vi "1_FindWorkingZDistancewPlaceholder.vi"(6 "Axis Speeds":T2, 7 "Focusing test interval [mm]":dbl, 8 "error in (no error)":errorcluster, 9 "Stepsize [mm]":dbl, 10 "Autofocus Coordinates":T3, 11 "Session in":T1) -> (0 "error out":errorcluster, 1 "Optimized working distance":dbl, 2 "XYZ Stage Current Position":T4, 3 "Session out":T1, 5 "Finished!":bool)   [LabVIEW 2016]
uses:
  <vilib>/userdefined/High Color/IMAQdx.ctl
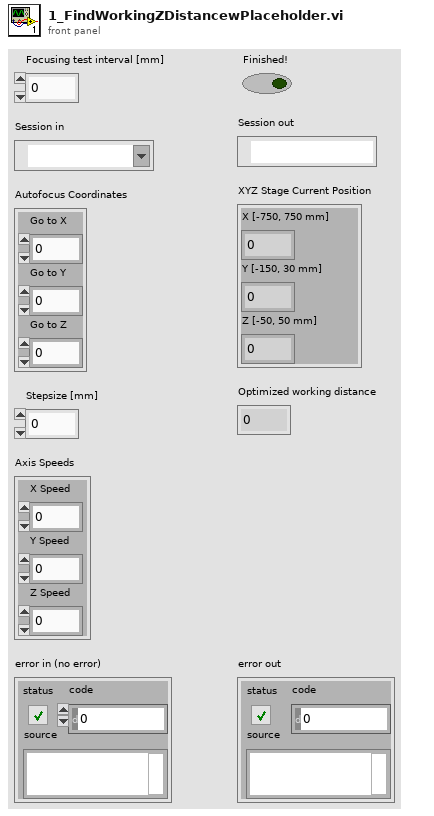
[diagram p1: front panel]
types:
  T1 = typedef "IMAQdx.ctl" = refnum<k21>
  T2 = cluster{"X Speed":dbl, "Y Speed":dbl, "Z Speed":dbl}
  T3 = cluster{"Go to X":dbl, "Go to Y":dbl, "Go to Z":dbl}
  T4 = cluster{"X [-750, 750 mm]":dbl, "Y [-150, 30 mm]":dbl, "Z [-50, 50 mm]":dbl}
  T5 = typedef "IMAQ Image.ctl" = refnum<image>
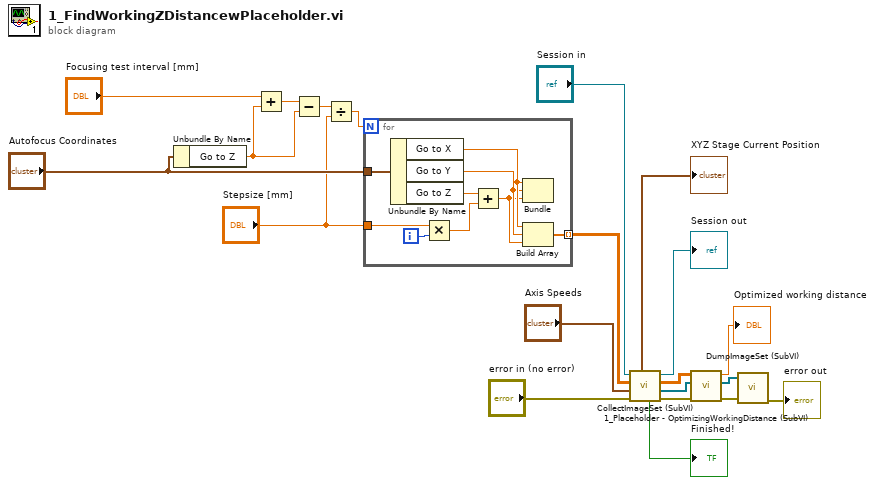
[diagram p0: block diagram]
diagram:
  n1 = Unbundle By Name("Autofocus Coordinates") -> ("Go to Z"=w17:dbl)
  n2 = Add(x="Focusing test interval [mm]", y=w17) -> (x+y=w16:dbl)
  n3 = Subtract(x=w16, y=w17) -> (x-y=w13:dbl)
  n4 = Divide(x=w13, y="Stepsize [mm]") -> (x/y=w14:dbl)
  n5 = for {
    N: w14 -> [_]
    tunnel: "Autofocus Coordinates" -> [w29]
    tunnel: [w25] -> w10 mode=indexing
    tunnel: "Stepsize [mm]" -> [w22]
    i -> [w23]
    n6 = Unbundle By Name(w29) -> ("Go to X"=w28:dbl, "Go to Y"=w27:dbl, "Go to Z"=w30:dbl)
    n7 = Multiply(x=w22, y=w23) -> (x*y=w24:dbl)
    n8 = Add(x=w30, y=w24) -> (x+y=w26:dbl)
    n9 = Bundle("Go to X"=w28, "Go to Y"=w27, w26) -> ()  [unwired: 1 in, 1 out]
    n10 = Build Array(w28, w27, w26) -> (w25:dbl[])
  }
  n11 = call "CollectImageSet (SubVI).vi"("error in"="error in (no error)", "Axes Speeds [mm/s]"="Axis Speeds", "Set of Coordinates to Process"=w10, "Session in"="Session in") -> ("error out"=w2:errorcluster, "Image Array"=w1:T5[], "Captured positions"=w3:dbl[][], "Session out"=→"Session out":T1, "Finished!"=→"Finished!":bool, "XYZ Stage Current Position"=→"XYZ Stage Current Position":T4)  [unwired: 2 in]
  n12 = call "1_Placeholder - OptimizingWorkingDistance (SubVI).vi"("error in (no error)"=w2, "Image Array in"=w1, "Captured positions"=w3) -> ("error out"=w7:errorcluster, "Image Array out"=w6:T5[], "Optimized working distance"=→"Optimized working distance":dbl)  [unwired: 6 in]
  n13 = call "DumpImageSet (SubVI).vi"("error in (no error)"=w7, "Calibrated Image Array"=w6) -> ("error out"=→"error out":errorcluster)  [unwired: 6 in]
